vi "FrozenFraction_Concatinate.vi"(1 "Freeze Fraction":dbl[][](array[numeric])) -> (0 "Freeze Fraction Concatinated":dbl[](array[numeric]))   [LabVIEW 2024]
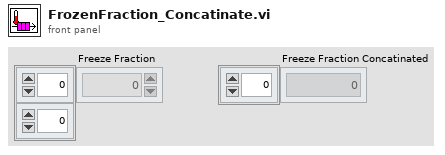
[diagram p1: front panel]
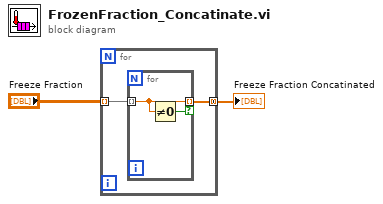
[diagram p0: block diagram]
diagram:
  n1 = for {
    tunnel: "Freeze Fraction" -> [w4] mode=indexing
    tunnel: [w3] -> w2 mode=concatenating
    n2 = for {
      tunnel: w4 -> [w5] mode=indexing
      tunnel: [w5] -> w3 mode=indexing if=w6
      n3 = Not Equal To 0?(x=w5) -> (x != 0?=w6:bool)
    }
  }
  "Freeze Fraction Concatinated" <- w2
